vi "black--constant.vi"() -> ()   [LabVIEW 2018, in "Resistor Band Colors.lvlib"]
uses:
  Resistor Band Colors.lvlib
panel:
  out "Negro":u32
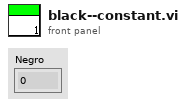
[diagram p1: front panel]
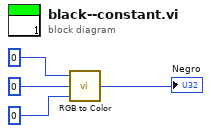
[diagram p0: block diagram]
diagram:
  n1 = call <vilib>:"RGB to Color.vi"("B"=u8 0 ("R"), "G"=u8 0 ("R"), "R"=u8 0) -> ("Color"=→"Negro":u32)
